vi "GetCalData.vi"(6 "Open new file T":bool, 7 "Ary In":dbl[][](array[numeric])=[[20000.0, -10.081], [20050.0, -10.248], [20100.0, -10.146], [20150.0, -10.499], [20200.0, -10.364], [20250.0, -10.204], [20300.0, -10.317], [20350.0, -10.223], [20400.0, -10.182], [20450.0, -10.2], [20500.0, -10.217], [20550.0, -10.208], [20600.0, -10.198], [20650.0, -10.242], [20700.0, -10.371], [20750.0, -10.383], [20800.0, -10.312], [20850.0, -10.405], [20900.0, -10.358], [20950.0, -10.357], [21000.0, -10.352], [21050.0, -10.375], [21100.0, -10.361], [21150.0, -10.358], [21200.0, -10.368], [21250.0, -10.414], [21300.0, -10.42], [21350.0, -10.405], [21400.0, -10.43], [21450.0, -10.476], [21500.0, -10.457], [21550.0, -10.591], [21600.0, -10.599], [21650.0, -10.534], [21700.0, -10.501], [21750.0, -10.549], [21800.0, -10.634], [21850.0, -10.636], [21900.0, -10.61], [21950.0, -10.649], [22000.0, -10.626], [22050.0, -10.694], [22100.0, -10.749], [22150.0, -10.652], [22200.0, -10.582], [22250.0, -10.661], [22300.0, -10.673], [22350.0, -10.755], [22400.0, -10.785], [22450.0, -10.737], [22500.0, -10.827], [22550.0, -10.799], [22600.0, -11.067], [22650.0, -10.932], [22700.0, -10.703], [22750.0, -10.853], [22800.0, -10.938], [22850.0, -10.939], [22900.0, -10.986], [22950.0, -10.93], [23000.0, -10.906], [23050.0, -10.934], [23100.0, -11.009], [23150.0, -11.179], [23200.0, -11.064], [23250.0, -10.98], [23300.0, -11.214], [23350.0, -11.153], [23400.0, -11.091], [23450.0, -11.127], [23500.0, -11.109], [23550.0, -11.121], [23600.0, -11.105], [23650.0, -11.133], [23700.0, -11.119], [23750.0, -11.116], [23800.0, -11.119], [23850.0, -11.273], [23900.0, -11.364], [23950.0, -11.233], [24000.0, -11.28], [24050.0, -11.236], [24100.0, -11.252], [24150.0, -11.232], [24200.0, -11.252], [24250.0, -11.289], [24300.0, -11.149], [24350.0, -11.184], [24400.0, -11.264], [24450.0, -11.344], [24500.0, -11.29], [24550.0, -11.33], [24600.0, -11.353], [24650.0, -11.334], [24700.0, -11.482], [24750.0, -11.449], [24800.0, -11.321], [24850.0, -11.338], [24900.0, -11.44], [24950.0, -11.497], [25000.0, -11.44], [25050.0, -11.47], [25100.0, -11.447], [25150.0, -11.456], [25200.0, -11.471], [25250.0, -11.632], [25300.0, -11.524], [25350.0, -11.565], [25400.0, -11.56], [25450.0, -11.656], [25500.0, -11.615], [25550.0, -11.651], [25600.0, -11.641], [25650.0, -11.727], [25700.0, -11.719], [25750.0, -11.768], [25800.0, -11.802], [25850.0, -11.731], [25900.0, -11.866], [25950.0, -11.763], [26000.0, -11.802], [26050.0, -11.811], [26100.0, -11.831], [26150.0, -11.766], [26200.0, -11.889], [26250.0, -11.923], [26300.0, -11.941], [26350.0, -11.973], [26400.0, -11.87], [26450.0, -11.947], [26500.0, -11.905], [26550.0, -11.927], [26600.0, -11.865], [26650.0, -11.85], [26700.0, -11.916], [26750.0, -11.823], [26800.0, -11.785], [26850.0, -11.9], [26900.0, -12.076], [26950.0, -11.883], [27000.0, -12.045], [27050.0, -11.891], [27100.0, -11.905], [27150.0, -11.951], [27200.0, -11.862], [27250.0, -11.912], [27300.0, -11.779], [27350.0, -11.837], [27400.0, -11.942], [27450.0, -11.956], [27500.0, -11.832], [27550.0, -11.946], [27600.0, -11.86], [27650.0, -11.884], [27700.0, -11.987], [27750.0, -11.877], [27800.0, -11.88], [27850.0, -11.876], [27900.0, -11.912], [27950.0, -11.926], [28000.0, -11.932], [28050.0, -11.954], [28100.0, -12.12], [28150.0, -11.94], [28200.0, -11.835], [28250.0, -11.881], [28300.0, -11.877], [28350.0, -11.877], [28400.0, -11.918], [28450.0, -11.961], [28500.0, -11.995], [28550.0, -12.068], [28600.0, -12.06], [28650.0, -12.102], [28700.0, -12.048], [28750.0, -11.978], [28800.0, -12.227], [28850.0, -12.191], [28900.0, -12.152], [28950.0, -12.124], [29000.0, -12.24], [29050.0, -12.206], [29100.0, -12.202], [29150.0, -12.247], [29200.0, -12.232], [29250.0, -12.455], [29300.0, -12.135], [29350.0, -12.274], [29400.0, -12.643], [29450.0, -12.698], [29500.0, -12.508], [29550.0, -12.691], [29600.0, -12.889], [29650.0, -12.436], [29700.0, -12.734], [29750.0, -12.443], [29800.0, -12.617], [29850.0, -12.47], [29900.0, -12.476], [29950.0, -13.271], [30000.0, -12.951], [30050.0, -12.719], [30100.0, -12.892], [30150.0, -13.317], [30200.0, -12.734], [30250.0, -13.113], [30300.0, -12.913], [30350.0, -12.965], [30400.0, -12.99], [30450.0, -12.751], [30500.0, -13.131], [30550.0, -12.798], [30600.0, -12.974], [30650.0, -12.875], [30700.0, -13.061], [30750.0, -13.116], [30800.0, -13.087], [30850.0, -13.313], [30900.0, -13.245], [30950.0, -13.432], [31000.0, -12.974], [31050.0, -13.228], [31100.0, -13.093], [31150.0, -13.102], [31200.0, -13.082], [31250.0, -13.019], [31300.0, -13.264], [31350.0, -13.029], [31400.0, -13.204], [31450.0, -13.134], [31500.0, -13.478], [31550.0, -13.028], [31600.0, -13.258], [31650.0, -13.22], [31700.0, -13.082], [31750.0, -13.263], [31800.0, -13.064], [31850.0, -13.28], [31900.0, -13.211], [31950.0, -13.074], [32000.0, -13.217], [32050.0, -13.238], [32100.0, -13.023], [32150.0, -13.128], [32200.0, -13.335], [32250.0, -13.139], [32300.0, -13.323], [32350.0, -13.155], [32400.0, -13.205], [32450.0, -13.332], [32500.0, -13.218], [32550.0, -13.332], [32600.0, -13.178], [32650.0, -13.236], [32700.0, -13.369], [32750.0, -13.26], [32800.0, -13.234], [32850.0, -13.242], [32900.0, -13.251], [32950.0, -13.285], [33000.0, -13.341], [33050.0, -13.354], [33100.0, -13.385], [33150.0, -13.44], [33200.0, -13.486], [33250.0, -13.422], [33300.0, -13.618], [33350.0, -13.468], [33400.0, -13.446], [33450.0, -13.41], [33500.0, -13.419], [33550.0, -13.431], [33600.0, -13.487], [33650.0, -13.57], [33700.0, -13.529], [33750.0, -13.813], [33800.0, -13.599], [33850.0, -13.954], [33900.0, -14.004], [33950.0, -13.841], [34000.0, -13.82], [34050.0, -13.724], [34100.0, -13.734], [34150.0, -13.678], [34200.0, -13.932], [34250.0, -13.765], [34300.0, -13.915], [34350.0, -13.771], [34400.0, -13.882], [34450.0, -14.169], [34500.0, -14.137], [34550.0, -14.097], [34600.0, -13.979], [34650.0, -14.217], [34700.0, -13.86], [34750.0, -14.08], [34800.0, -14.004], [34850.0, -13.992], [34900.0, -13.909], [34950.0, -13.973], [35000.0, -13.981], [35050.0, -14.02], [35100.0, -14.182], [35150.0, -13.971], [35200.0, -14.168], [35250.0, -13.979], [35300.0, -14.029], [35350.0, -14.096], [35400.0, -14.033], [35450.0, -14.069], [35500.0, -14.033], [35550.0, -14.019], [35600.0, -14.011], [35650.0, -14.083], [35700.0, -14.006], [35750.0, -14.039], [35800.0, -14.001], [35850.0, -14.038], [35900.0, -14.074], [35950.0, -14.096], [36000.0, -14.3], [36050.0, -14.197], [36100.0, -14.194], [36150.0, -14.219], [36200.0, -14.268], [36250.0, -14.255], [36300.0, -14.407], [36350.0, -14.254], [36400.0, -14.275], [36450.0, -14.422], [36500.0, -14.383], [36550.0, -14.518], [36600.0, -14.583], [36650.0, -14.561], [36700.0, -14.665], [36750.0, -14.707], [36800.0, -14.683], [36850.0, -14.833], [36900.0, -14.84], [36950.0, -14.805], [37000.0, -15.016], [37050.0, -14.98], [37100.0, -14.815], [37150.0, -14.922], [37200.0, -14.918], [37250.0, -14.943], [37300.0, -14.912], [37350.0, -14.925], [37400.0, -15.021], [37450.0, -14.969], [37500.0, -14.985], [37550.0, -14.984], [37600.0, -15.169], [37650.0, -15.022], [37700.0, -14.972], [37750.0, -15.115], [37800.0, -15.157], [37850.0, -14.903], [37900.0, -14.922], [37950.0, -14.917], [38000.0, -14.892], [38050.0, -14.928], [38100.0, -14.916], [38150.0, -15.062], [38200.0, -14.892], [38250.0, -14.919], [38300.0, -14.932], [38350.0, -14.973], [38400.0, -14.973], [38450.0, -14.879], [38500.0, -14.861], [38550.0, -14.801], [38600.0, -14.85], [38650.0, -14.946], [38700.0, -14.847], [38750.0, -14.798], [38800.0, -14.84], [38850.0, -14.892], [38900.0, -14.92], [38950.0, -14.96], [39000.0, -14.897], [39050.0, -14.885], [39100.0, -14.916], [39150.0, -15.135], [39200.0, -15.276], [39250.0, -15.047], [39300.0, -15.112], [39350.0, -15.07], [39400.0, -15.18], [39450.0, -15.381], [39500.0, -15.118], [39550.0, -15.065], [39600.0, -15.085], [39650.0, -15.133], [39700.0, -15.267], [39750.0, -15.334], [39800.0, -15.441], [39850.0, -15.319], [39900.0, -15.307], [39950.0, -15.616], [40000.0, -15.84]], 8 "error in (no error)":errorcluster, 9 "RF Freq (MHz)":dbl=40000.0, 10 "DeleteHeader(t)":bool, 11 "cal file path (dialog if empty)":path=path "C:/RageATE/Automated Tests/Tetra WAM/PRODUCTION/Test Benches/Common/Horn_Gain_121322-2.csv") -> (0 "error out":errorcluster, 1 "Ampl Out":dbl=-15.84, 2 "Cal Freq Out":dbl=40000.0, 3 "cal file path out":path=path "C:/RageATE/Automated Tests/Tetra WAM/PRODUCTION/Test Benches/Common/Horn_Gain_121322-2.csv", 4 "Coerced(T)":bool, 5 "array out":dbl[][](array[numeric])=[[20000.0, -10.081], [20050.0, -10.248], [20100.0, -10.146], [20150.0, -10.499], [20200.0, -10.364], [20250.0, -10.204], [20300.0, -10.317], [20350.0, -10.223], [20400.0, -10.182], [20450.0, -10.2], [20500.0, -10.217], [20550.0, -10.208], [20600.0, -10.198], [20650.0, -10.242], [20700.0, -10.371], [20750.0, -10.383], [20800.0, -10.312], [20850.0, -10.405], [20900.0, -10.358], [20950.0, -10.357], [21000.0, -10.352], [21050.0, -10.375], [21100.0, -10.361], [21150.0, -10.358], [21200.0, -10.368], [21250.0, -10.414], [21300.0, -10.42], [21350.0, -10.405], [21400.0, -10.43], [21450.0, -10.476], [21500.0, -10.457], [21550.0, -10.591], [21600.0, -10.599], [21650.0, -10.534], [21700.0, -10.501], [21750.0, -10.549], [21800.0, -10.634], [21850.0, -10.636], [21900.0, -10.61], [21950.0, -10.649], [22000.0, -10.626], [22050.0, -10.694], [22100.0, -10.749], [22150.0, -10.652], [22200.0, -10.582], [22250.0, -10.661], [22300.0, -10.673], [22350.0, -10.755], [22400.0, -10.785], [22450.0, -10.737], [22500.0, -10.827], [22550.0, -10.799], [22600.0, -11.067], [22650.0, -10.932], [22700.0, -10.703], [22750.0, -10.853], [22800.0, -10.938], [22850.0, -10.939], [22900.0, -10.986], [22950.0, -10.93], [23000.0, -10.906], [23050.0, -10.934], [23100.0, -11.009], [23150.0, -11.179], [23200.0, -11.064], [23250.0, -10.98], [23300.0, -11.214], [23350.0, -11.153], [23400.0, -11.091], [23450.0, -11.127], [23500.0, -11.109], [23550.0, -11.121], [23600.0, -11.105], [23650.0, -11.133], [23700.0, -11.119], [23750.0, -11.116], [23800.0, -11.119], [23850.0, -11.273], [23900.0, -11.364], [23950.0, -11.233], [24000.0, -11.28], [24050.0, -11.236], [24100.0, -11.252], [24150.0, -11.232], [24200.0, -11.252], [24250.0, -11.289], [24300.0, -11.149], [24350.0, -11.184], [24400.0, -11.264], [24450.0, -11.344], [24500.0, -11.29], [24550.0, -11.33], [24600.0, -11.353], [24650.0, -11.334], [24700.0, -11.482], [24750.0, -11.449], [24800.0, -11.321], [24850.0, -11.338], [24900.0, -11.44], [24950.0, -11.497], [25000.0, -11.44], [25050.0, -11.47], [25100.0, -11.447], [25150.0, -11.456], [25200.0, -11.471], [25250.0, -11.632], [25300.0, -11.524], [25350.0, -11.565], [25400.0, -11.56], [25450.0, -11.656], [25500.0, -11.615], [25550.0, -11.651], [25600.0, -11.641], [25650.0, -11.727], [25700.0, -11.719], [25750.0, -11.768], [25800.0, -11.802], [25850.0, -11.731], [25900.0, -11.866], [25950.0, -11.763], [26000.0, -11.802], [26050.0, -11.811], [26100.0, -11.831], [26150.0, -11.766], [26200.0, -11.889], [26250.0, -11.923], [26300.0, -11.941], [26350.0, -11.973], [26400.0, -11.87], [26450.0, -11.947], [26500.0, -11.905], [26550.0, -11.927], [26600.0, -11.865], [26650.0, -11.85], [26700.0, -11.916], [26750.0, -11.823], [26800.0, -11.785], [26850.0, -11.9], [26900.0, -12.076], [26950.0, -11.883], [27000.0, -12.045], [27050.0, -11.891], [27100.0, -11.905], [27150.0, -11.951], [27200.0, -11.862], [27250.0, -11.912], [27300.0, -11.779], [27350.0, -11.837], [27400.0, -11.942], [27450.0, -11.956], [27500.0, -11.832], [27550.0, -11.946], [27600.0, -11.86], [27650.0, -11.884], [27700.0, -11.987], [27750.0, -11.877], [27800.0, -11.88], [27850.0, -11.876], [27900.0, -11.912], [27950.0, -11.926], [28000.0, -11.932], [28050.0, -11.954], [28100.0, -12.12], [28150.0, -11.94], [28200.0, -11.835], [28250.0, -11.881], [28300.0, -11.877], [28350.0, -11.877], [28400.0, -11.918], [28450.0, -11.961], [28500.0, -11.995], [28550.0, -12.068], [28600.0, -12.06], [28650.0, -12.102], [28700.0, -12.048], [28750.0, -11.978], [28800.0, -12.227], [28850.0, -12.191], [28900.0, -12.152], [28950.0, -12.124], [29000.0, -12.24], [29050.0, -12.206], [29100.0, -12.202], [29150.0, -12.247], [29200.0, -12.232], [29250.0, -12.455], [29300.0, -12.135], [29350.0, -12.274], [29400.0, -12.643], [29450.0, -12.698], [29500.0, -12.508], [29550.0, -12.691], [29600.0, -12.889], [29650.0, -12.436], [29700.0, -12.734], [29750.0, -12.443], [29800.0, -12.617], [29850.0, -12.47], [29900.0, -12.476], [29950.0, -13.271], [30000.0, -12.951], [30050.0, -12.719], [30100.0, -12.892], [30150.0, -13.317], [30200.0, -12.734], [30250.0, -13.113], [30300.0, -12.913], [30350.0, -12.965], [30400.0, -12.99], [30450.0, -12.751], [30500.0, -13.131], [30550.0, -12.798], [30600.0, -12.974], [30650.0, -12.875], [30700.0, -13.061], [30750.0, -13.116], [30800.0, -13.087], [30850.0, -13.313], [30900.0, -13.245], [30950.0, -13.432], [31000.0, -12.974], [31050.0, -13.228], [31100.0, -13.093], [31150.0, -13.102], [31200.0, -13.082], [31250.0, -13.019], [31300.0, -13.264], [31350.0, -13.029], [31400.0, -13.204], [31450.0, -13.134], [31500.0, -13.478], [31550.0, -13.028], [31600.0, -13.258], [31650.0, -13.22], [31700.0, -13.082], [31750.0, -13.263], [31800.0, -13.064], [31850.0, -13.28], [31900.0, -13.211], [31950.0, -13.074], [32000.0, -13.217], [32050.0, -13.238], [32100.0, -13.023], [32150.0, -13.128], [32200.0, -13.335], [32250.0, -13.139], [32300.0, -13.323], [32350.0, -13.155], [32400.0, -13.205], [32450.0, -13.332], [32500.0, -13.218], [32550.0, -13.332], [32600.0, -13.178], [32650.0, -13.236], [32700.0, -13.369], [32750.0, -13.26], [32800.0, -13.234], [32850.0, -13.242], [32900.0, -13.251], [32950.0, -13.285], [33000.0, -13.341], [33050.0, -13.354], [33100.0, -13.385], [33150.0, -13.44], [33200.0, -13.486], [33250.0, -13.422], [33300.0, -13.618], [33350.0, -13.468], [33400.0, -13.446], [33450.0, -13.41], [33500.0, -13.419], [33550.0, -13.431], [33600.0, -13.487], [33650.0, -13.57], [33700.0, -13.529], [33750.0, -13.813], [33800.0, -13.599], [33850.0, -13.954], [33900.0, -14.004], [33950.0, -13.841], [34000.0, -13.82], [34050.0, -13.724], [34100.0, -13.734], [34150.0, -13.678], [34200.0, -13.932], [34250.0, -13.765], [34300.0, -13.915], [34350.0, -13.771], [34400.0, -13.882], [34450.0, -14.169], [34500.0, -14.137], [34550.0, -14.097], [34600.0, -13.979], [34650.0, -14.217], [34700.0, -13.86], [34750.0, -14.08], [34800.0, -14.004], [34850.0, -13.992], [34900.0, -13.909], [34950.0, -13.973], [35000.0, -13.981], [35050.0, -14.02], [35100.0, -14.182], [35150.0, -13.971], [35200.0, -14.168], [35250.0, -13.979], [35300.0, -14.029], [35350.0, -14.096], [35400.0, -14.033], [35450.0, -14.069], [35500.0, -14.033], [35550.0, -14.019], [35600.0, -14.011], [35650.0, -14.083], [35700.0, -14.006], [35750.0, -14.039], [35800.0, -14.001], [35850.0, -14.038], [35900.0, -14.074], [35950.0, -14.096], [36000.0, -14.3], [36050.0, -14.197], [36100.0, -14.194], [36150.0, -14.219], [36200.0, -14.268], [36250.0, -14.255], [36300.0, -14.407], [36350.0, -14.254], [36400.0, -14.275], [36450.0, -14.422], [36500.0, -14.383], [36550.0, -14.518], [36600.0, -14.583], [36650.0, -14.561], [36700.0, -14.665], [36750.0, -14.707], [36800.0, -14.683], [36850.0, -14.833], [36900.0, -14.84], [36950.0, -14.805], [37000.0, -15.016], [37050.0, -14.98], [37100.0, -14.815], [37150.0, -14.922], [37200.0, -14.918], [37250.0, -14.943], [37300.0, -14.912], [37350.0, -14.925], [37400.0, -15.021], [37450.0, -14.969], [37500.0, -14.985], [37550.0, -14.984], [37600.0, -15.169], [37650.0, -15.022], [37700.0, -14.972], [37750.0, -15.115], [37800.0, -15.157], [37850.0, -14.903], [37900.0, -14.922], [37950.0, -14.917], [38000.0, -14.892], [38050.0, -14.928], [38100.0, -14.916], [38150.0, -15.062], [38200.0, -14.892], [38250.0, -14.919], [38300.0, -14.932], [38350.0, -14.973], [38400.0, -14.973], [38450.0, -14.879], [38500.0, -14.861], [38550.0, -14.801], [38600.0, -14.85], [38650.0, -14.946], [38700.0, -14.847], [38750.0, -14.798], [38800.0, -14.84], [38850.0, -14.892], [38900.0, -14.92], [38950.0, -14.96], [39000.0, -14.897], [39050.0, -14.885], [39100.0, -14.916], [39150.0, -15.135], [39200.0, -15.276], [39250.0, -15.047], [39300.0, -15.112], [39350.0, -15.07], [39400.0, -15.18], [39450.0, -15.381], [39500.0, -15.118], [39550.0, -15.065], [39600.0, -15.085], [39650.0, -15.133], [39700.0, -15.267], [39750.0, -15.334], [39800.0, -15.441], [39850.0, -15.319], [39900.0, -15.307], [39950.0, -15.616], [40000.0, -15.84]])   [LabVIEW 2018]
uses:
  <vilib>/Utility/file.llb/Read Delimited Spreadsheet (string).vi
panel:
  out "name":string="WAM_NF_MASK.txt"
  out "stripped path":path=path "C:/RageATE/Automated Tests/Tetra WAM/DVT"
  # "This Vi takes in a csv file  [Freq(MHz),Ampl (dBm)]\n1. Scans the freq column (0) for a match\n2. If no match will find closest frequency\n3. Reports the Amplitude (column 1)\n4. Reports the frequency that the search was coerced to and whether or not there was coersion"
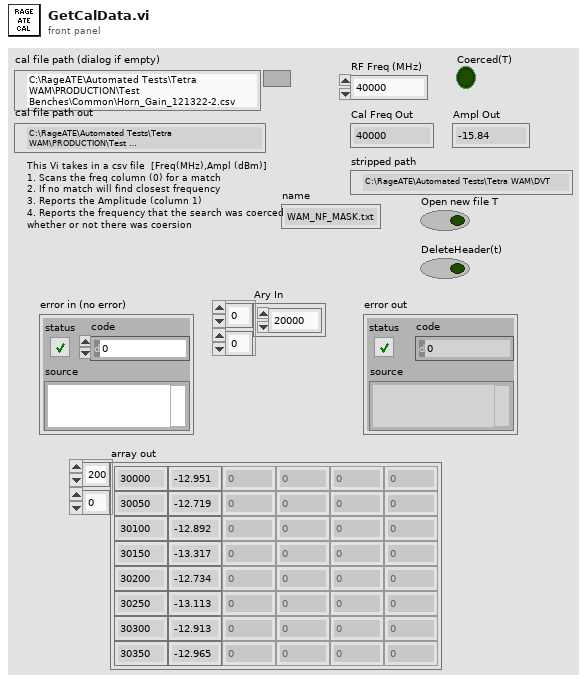
[diagram p1: front panel]
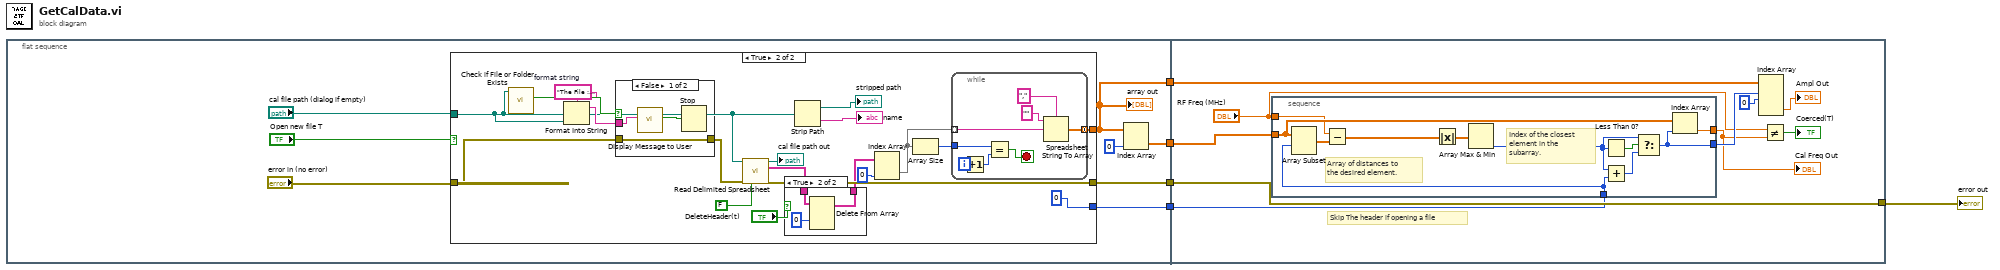
[diagram p0: block diagram]
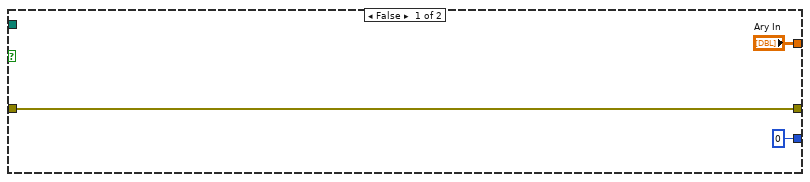
[diagram p2: hidden frame]
diagram:
  n1 = flat-sequence {
    tunnel: [w12] -> w5
    tunnel: [w7] -> w4
    tunnel: [w10] -> w3
    tunnel: [w9] -> w1
    tunnel: w5 -> [w61]
    tunnel: w4 -> [w60]
    tunnel: w3 -> [w53]
    tunnel: [w53] -> w2
    tunnel: w1 -> [w52]
    frame #0 {
      n2 = case shown="True" "Open new file T" {
        tunnel: ["Ary In" w31] -> w7
        tunnel: "error in (no error)" -> [w15 w18]
        tunnel: [w15 w30] -> w10
        tunnel: [0 ("start index (0)") 0 ("start index (0)")] -> w9
        tunnel: "cal file path (dialog if empty)" -> [_ w19]
        frame False {
        }
        frame True {
          w20 = "The File : %s cant be located . Aborting"  # format string
          n3 = call <vilib>:"Check if File or Folder Exists.vi"("path"=w19) -> ("file or folder exists?"=w22:bool)  [unwired: 8 in, 2 out]
          n4 = Format Into String(format string=w20, w19) -> (resulting string=w21:string)  [unwired: 2 in, 1 out]
          n5 = case shown="False" w22 {
            tunnel: w21 -> [w38 _]
            tunnel: w18 -> [w36 w39]
            tunnel: [w36 w39] -> w17
            frame False {
              n6 = call "Display Message to User"("Message"=w38) -> ("OK"=w37:bool)  [unwired: 9 in, 1 out]
              n7 = Stop(stop? (T)=w37) -> ()
            }
            frame True {
            }
          }
          n8 = call-poly <vilib>:"Read Delimited Spreadsheet.vi"("file path (dialog if empty)"=w19, "error in (no error)"=w17, "transpose? (F)"=FALSE) -> ("new file path (Not A Path if cancelled)"=→"cal file path out":path, "all rows"=w25:string[][], "error out"=w30:errorcluster)  [unwired: 7 in, 3 out]
          n9 = case shown="True" "DeleteHeader(t)" {
            tunnel: w25 -> [w40 w43]
            tunnel: [w40 w42] -> w24
            frame False {
            }
            frame True {
              n10 = Delete From Array(array=w43, index (row)=0) -> (array with subset deleted=w42:string[][])  [unwired: 2 in, 1 out]
            }
          }
          n11 = Strip Path(path=w19) -> (stripped path=→"stripped path":path, name=→"name":string)
          n12 = Index Array(array=w24, index (col)=0 ("disabled index (col)")) -> (element=w33:string[])  [unwired: 1 in]
          n13 = Array Size(array=w33) -> (size(s)=w32:i32)
          n14 = while {
            tunnel: w33 -> [w51] mode=indexing
            tunnel: w32 -> [w48]
            tunnel: [w45] -> w31 mode=concatenating
            i -> [w50]
            stop <- w49 stop-if-true
            n15 = Increment(x=w50) -> (x+1=w44:i32)
            n16 = Equal?(x=w48, y=w44) -> (x = y?=w49:bool)
            n17 = Spreadsheet String To Array(delimiter (Tab)=",", format string="", spreadsheet string=w51) -> (array=w45:dbl[][])  [unwired: 1 in]
          }
        }
      }
      "array out" <- w7
      n18 = Index Array(array=w7, index (col)=0 ("disabled index (col)")) -> (element=w12:dbl[])  [unwired: 1 in]
    }
    frame #1 {
      # "Skip The header if opening a file"
      n19 = stacked-sequence {
        tunnel: [w72] -> w59
        tunnel: [w64] -> w56
        tunnel: "RF Freq (MHz)" -> [w69]
        tunnel: w61 -> [w71]
        tunnel: w52 -> [w62]
        frame #0 {
          # "Index of the closest element in the subarray."
          # "Array of distances to the desired element."
          n20 = Array Subset(array=w71, index=w62) -> (w70:dbl[])  [unwired: 1 in]
          n21 = Subtract(x=w69, y=w70) -> (x-y=w63:dbl[])
          n22 = Absolute Value(x=w63) -> (abs(x)=w65:dbl[])
          n23 = Array Max & Min(array=w65) -> (min index (indices)=w67:i32)  [unwired: 3 out]
          n24 = Less Than 0?(x=w67) -> (x < 0?=w66:bool)
          n25 = Add(x=w67, y=w62) -> (x+y=w68:i32)
          n26 = Select(t=w67, s=w66, f=w68) -> (s? t:f=w72:i32)
          n27 = Index Array(array=w71, index=w72) -> (element=w64:dbl)
        }
      }
      "Cal Freq Out" <- w56
      n28 = Index Array(array=w60, index (row) #1=w59, index (col) #1=0 ("disabled index (col)")) -> (element #2=→"Ampl Out":dbl)  [unwired: 2 in, 1 out]
      n29 = Not Equal?(x="RF Freq (MHz)", y=w56) -> (x != y?=→"Coerced(T)":bool)
    }
  }
  "error out" <- w2
